vi "niFpgaPID_PIStatelessCore.vi"(0 "errors":T3 {"error" step=0.125}, 1 "reset? (F)":bool, 5 "enable bumpless transfer? (F)":bool, 7 "manual control":T6, 11 "state in":T2, 12 "gains":T4 {"proportional gain" step=0.125}, 13 "output range":T5={"output high (Inf)"=inf, "output low (-Inf)"=-inf}) -> (4 "output":sgl, 6 "error":sgl, 8 "actions":T1, 15 "state out":T2)   [LabVIEW 2020]
uses:
  <vilib>/rvi/Analysis/control/PID/Typedef/niFpgaPID_ManualControl.ctl
  <vilib>/rvi/Analysis/control/PID/Typedef/niFpgaPID_OutputRange.ctl
  <vilib>/rvi/Analysis/control/PID/Typedef/niFpgaPID_PIGains.ctl
  <vilib>/rvi/Analysis/control/PID/Typedef/niFpgaPID_PIErrors.ctl
  <vilib>/rvi/Analysis/control/PID/Typedef/niFpgaPID_PIState.ctl
  <vilib>/rvi/Analysis/control/PID/Typedef/niFpgaPID_PIActions.ctl
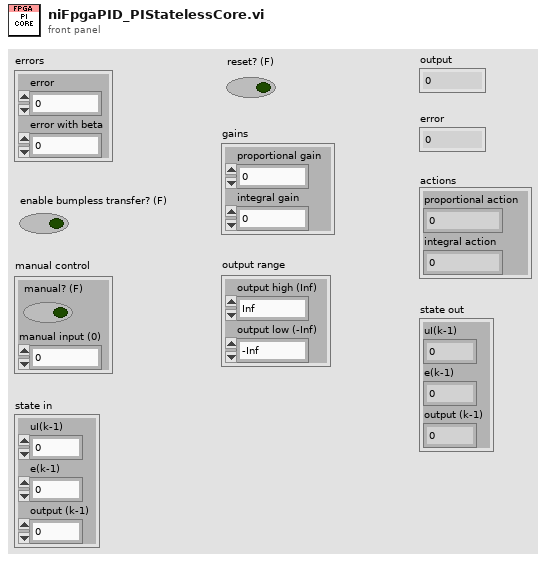
[diagram p1: front panel]
types:
  T1 = typedef "niFpgaPID_PIActions.ctl" = cluster{"proportional action":sgl, "integral action":sgl}
  T2 = typedef "niFpgaPID_PIState.ctl" = cluster{"uI(k-1)":sgl, "e(k-1)":sgl, "output (k-1)":sgl}
  T3 = typedef "niFpgaPID_PIErrors.ctl" = cluster{"error":sgl, "error with beta":sgl}
  T4 = typedef "niFpgaPID_PIGains.ctl" = cluster{"proportional gain":sgl, "integral gain":sgl}
  T5 = typedef "niFpgaPID_OutputRange.ctl" = cluster{"output high (Inf)":sgl, "output low (-Inf)":sgl}
  T6 = typedef "niFpgaPID_ManualControl.ctl" = cluster{"manual? (F)":bool, "manual input (0)":sgl}
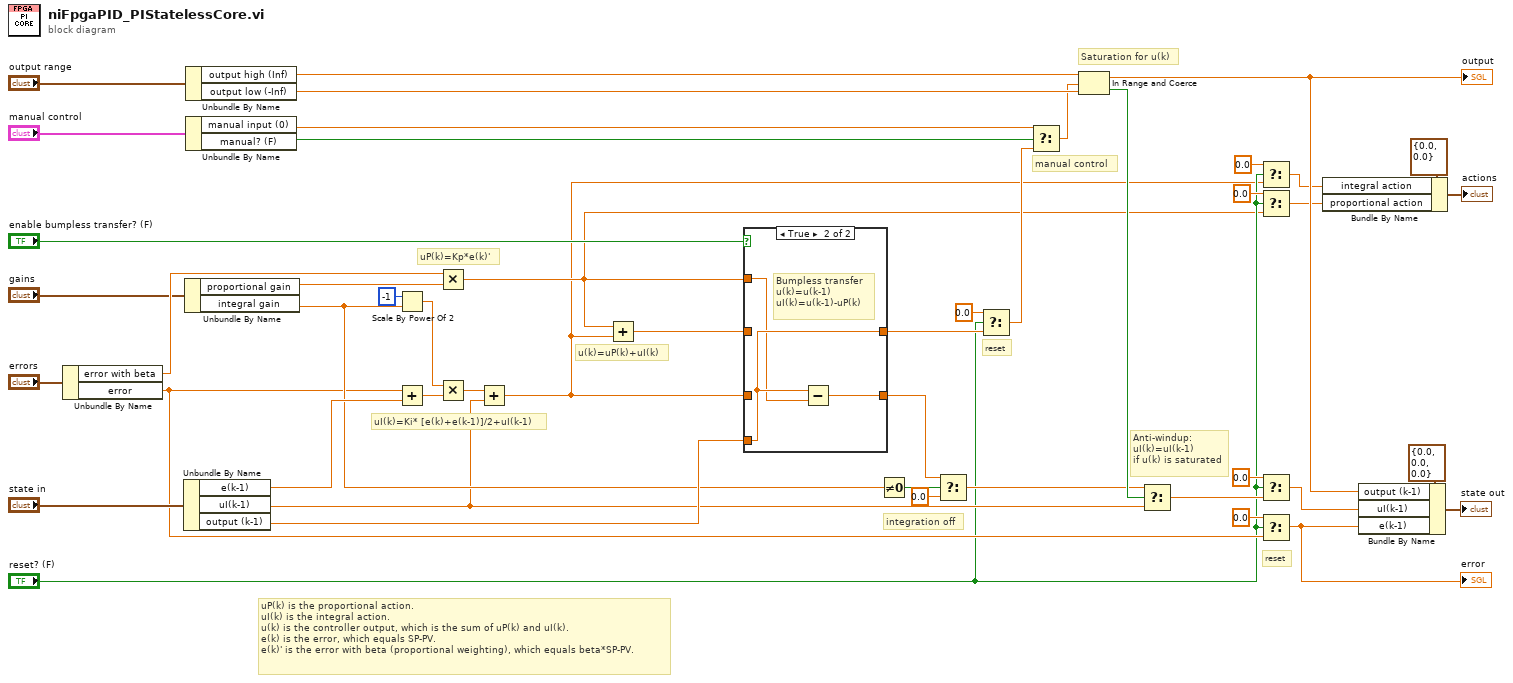
[diagram p0: block diagram]
diagram:
  # "uP(k) is the proportional action.\nuI(k) is the integral action.\nu(k) is the controller output, which is the sum of uP(k) and uI(k).\ne(k) is the error, which equals SP-PV.\ne(k)' is the error with beta (proportional weighting), which equals beta*SP-PV."
  # "integration off"
  # "reset"
  # "manual control"
  # "reset"
  # "Anti-windup:\nuI(k)=uI(k-1) \nif u(k) is saturated"
  # "Saturation for u(k)"
  # "u(k)=uP(k)+uI(k)"
  # "uI(k)=Ki* [e(k)+e(k-1)]/2+uI(k-1)"
  # "uP(k)=Kp*e(k)'"
  n1 = Unbundle By Name("errors") -> ("error with beta"=w43:sgl, "error"=w11:sgl)
  n2 = Unbundle By Name("state in") -> ("e(k-1)"=w33:sgl, "uI(k-1)"=w6:sgl, "output (k-1)"=w34:sgl)
  n3 = Unbundle By Name("gains") -> ("proportional gain"=w44:sgl, "integral gain"=w31:sgl)
  n4 = Unbundle By Name("output range") -> ("output high (Inf)"=w19:sgl, "output low (-Inf)"=w18:sgl)
  n5 = Unbundle By Name("manual control") -> ("manual input (0)"=w29:sgl, "manual? (F)"=w28:bool)
  n6 = Scale By Power Of 2(n=i16 -1, x=w31) -> (x*2^n=w40:sgl)
  n7 = Add(x=w11, y=w33) -> (x+y=w41:sgl)
  n8 = Multiply(x=w43, y=w44) -> (x*y=w2:sgl)
  n9 = Multiply(x=w40, y=w41) -> (x*y=w48:sgl)
  n10 = Add(x=w48, y=w6) -> (x+y=w1:sgl)
  n11 = Add(x=w2, y=w1) -> (x+y=w20:sgl)
  n12 = case shown="True" "enable bumpless transfer? (F)" {
    tunnel: w20 -> [w50 _]
    tunnel: [w50 w52] -> w25
    tunnel: w1 -> [w49 _]
    tunnel: [w49 w53] -> w27
    tunnel: w2 -> [_ w51]
    tunnel: w34 -> [_ w52]
    frame False {
    }
    frame True {
      # "Bumpless transfer\nu(k)=u(k-1)\nuI(k)=u(k-1)-uP(k)"
      n13 = Subtract(x=w52, y=w51) -> (x-y=w53:sgl)
    }
  }
  n14 = Not Equal To 0?(x=w31) -> (x != 0?=w32:bool)
  n15 = Select(t=w27, s=w32, f=sgl 0.0) -> (s? t:f=w7:sgl)
  n16 = Select(t=sgl 0.0 ("f"), s="reset? (F)", f=w25) -> (s? t:f=w24:sgl)
  n17 = Select(t=w29, s=w28, f=w24) -> (s? t:f=w17:sgl)
  n18 = In Range and Coerce(upper limit=w19, x=w17, lower limit=w18) -> (coerced(x)=w16:sgl, In Range?=w21:bool)
  "output" <- w16
  n19 = Select(t=w7, s=w21, f=w6) -> (s? t:f=w8:sgl)
  n20 = Select(t=sgl 0.0, s="reset? (F)", f=w1) -> (s? t:f=w12:sgl)
  n21 = Select(t=sgl 0.0, s="reset? (F)", f=w2) -> (s? t:f=w13:sgl)
  n22 = Select(t=sgl 0.0, s="reset? (F)", f=w8) -> (s? t:f=w5:sgl)
  n23 = Select(t=sgl 0.0, s="reset? (F)", f=w11) -> (s? t:f=w3:sgl)
  "error" <- w3
  n24 = Bundle By Name(cluster=T1 {"proportional action"=0.0, "integral action"=0.0} ("actions"), "integral action"=w12, "proportional action"=w13) -> (→"actions":T1)
  n25 = Bundle By Name(cluster=T2 {"uI(k-1)"=0.0, "e(k-1)"=0.0, "output (k-1)"=0.0} ("state out"), "output (k-1)"=w16, "uI(k-1)"=w5, "e(k-1)"=w3) -> (→"state out":T2)
